vi "Bertta_v09_9.vi"() -> ()   [LabVIEW 2015]
panel:
  out "element":bool
  out "Started:":string
  in  "SHUTDOWN":bool
  in  "MASTER CONTROL":bool
  in  "Tab Control":T1(tab)
  out "Output File":path caption="selected path"
  in  "Browse folder":path=path "" caption="start path"
  in  "Read Seq":bool
  in  "Save Seq":bool
  in  "Configuration file":path=path "C:/Users/shresplab/Desktop/BerttaConfiguration.lvm" caption="Filename"
  in  "OK Button 2":bool
  out "Boolean":bool
  in  "User (initials)":string
  in  "Project name":string
  in  "Description":string
  out "PUMP1":bool
  out "Target amount":dbl
  out "Scale weight":dbl
  out "Amount now":dbl
  out "Flow rate":dbl
  out "Time to target":dbl format="%<%H:%M:%S>t"
  out "Current step":dbl
  out "Target":dbl
  out "Amount now":dbl
  out "Amount now":dbl
  out "Target":dbl
  out "Current step":dbl
  out "Time to target":dbl format="%<%H:%M:%S>t"
  out "Flow rate":dbl
  out "Amount now":dbl
  out "Scale weight":dbl
  out "Target amount":dbl
  out "PUMP2":bool
  out "Sensor OK 6":bool
  out "Sensor OK 5":bool
  out "Sensor OK 4":bool
  out "Sensor OK 3":bool
  in  "OK Button":bool
  in  "Add comment":string
  out "PUMP3":bool
  out "Target amount":dbl
  out "Scale weight":dbl
  out "Amount now":dbl
  out "Flow rate":dbl
  out "Time to target":dbl format="%<%H:%M:%S>t"
  out "Current step":dbl
  out "Target":dbl
  out "Amount now":dbl
  out "Tr":dbl
  out "Tj in":dbl
  out "Tj out":dbl
  out "T set":dbl
  out "Current step":i32
  out "RPM":dbl
  out "Torque 2":dbl
  out "Waveform Chart 5":dynamicdata(graph)
  out "Waveform Chart 6":dynamicdata(graph)
  out "Waveform Chart 7":dynamicdata(graph)
  in  "Tab Control 2":T2(tab)
  out "Waveform Chart 3":dynamicdata(graph)
  out "Waveform Chart 8":dynamicdata(graph)
  out "Waveform Chart 11":dynamicdata(graph)
  out "Waveform Chart 13":dynamicdata(graph)
  out "Waveform Chart 9":dynamicdata(graph)
  out "Table":string[][](table)=[["14.8.2017 18.06.59", "0,000000", "417,670000", "-0,150000", "1,000000", "22,220000", "23,366837", "23,574959", "23,985852", "23,690000", "240,000000", "4,000000", "0,000000", "397,000000", "-397,000000", "1,000000"], ["14.8.2017 18.07.06", "0,000000", "417,640000", "-0,120000", "1,000000", "22,220000", "23,763115", "23,906257", "23,985694", "23,680000", "240,000000", "4,000000", "0,000000", "397,000000", "-397,000000", "1,000000"], ["14.8.2017 18.07.13", "0,000000", "417,640000", "-0,120000", "1,000000", "22,220000", "23,965922", "24,013440", "23,984906", "23,670000", "240,000000", "4,100000", "3,000000", "397,000000", "-397,000000", "1,000000"], ["14.8.2017 18.07.21", "0,000000", "417,640000", "-0,120000", "1,000000", "22,220000", "23,943860", "23,900110", "23,987113", "23,670000", "240,000000", "4,000000", "0,000000", "397,000000", "-397,000000", "1,000000"], ["14.8.2017 18.07.28", "0,000000", "417,640000", "-0,120000", "1,000000", "22,220000", "23,736328", "23,600018", "23,989004", "23,660000", "240,000000", "4,000000", "0,000000", "397,000000", "-397,000000", "1,000000"], ["14.8.2017 18.07.36", "0,000000", "417,640000", "-0,120000", "1,000000", "22,220000", "23,480910", "23,324538", "23,991053", "23,660000", "240,000000", "4,000000", "0,000000", "397,000000", "-397,000000", "1,000000"], ["14.8.2017 18.07.43", "0,000000", "417,640000", "-0,120000", "2,000000", "22,220000", "23,195579", "23,008270", "23,999093", "23,650000", "240,000000", "4,000000", "0,000000", "397,000000", "-397,000000", "1,000000"], ["14.8.2017 18.07.51", "0,000000", "417,650000", "-417,650000", "1,000000", "22,220000", "22,862541", "22,649021", "24,003979", "23,650000", "240,000000", "4,000000", "0,000000", "397,000000", "-397,000000", "2,000000"], ["14.8.2017 18.07.58", "0,000000", "417,640000", "0,010000", "1,000000", "22,220000", "22,541353", "22,354878", "24,005398", "23,650000", "240,000000", "4,000000", "0,000000", "397,000000", "-397,000000", "1,000000"], ["14.8.2017 18.08.06", "0,000000", "417,640000", "0,010000", "1,000000", "22,220000", "22,347931", "22,253738", "24,007605", "23,640000", "240,000000", "4,100000", "0,000000", "397,000000", "-397,000000", "1,000000"], ["14.8.2017 18.08.13", "0,000000", "417,640000", "0,010000", "1,000000", "22,220000", "22,329030", "22,302102", "24,006028", "23,640000", "240,000000", "4,000000", "0,000000", "395,820000", "-395,820000", "1,000000"], ["14.8.2017 18.08.20", "0,000000", "417,640000", "0,010000", "1,000000", "22,220000", "22,466849", "22,511320", "24,002403", "23,630000", "240,000000", "4,000000", "0,000000", "395,830000", "-0,010000", "1,000000"], ["14.8.2017 18.08.28", "0,000000", "417,640000", "0,010000", "1,000000", "22,220000", "22,707062", "22,835101", "24,000984", "23,620000", "240,000000", "4,000000", "0,000000", "395,830000", "-0,010000", "1,000000"], ["14.8.2017 18.08.35", "0,000000", "417,640000", "0,010000", "1,000000", "22,220000", "23,054104", "23,232979", "24,001299", "23,600000", "240,000000", "4,000000", "0,000000", "395,830000", "-0,010000", "1,000000"], ["14.8.2017 18.08.43", "0,000000", "417,640000", "0,010000", "1,000000", "22,220000", "23,412371", "23,522793", "24,002560", "23,590000", "240,000000", "4,000000", "0,000000", "395,820000", "0,000000", "1,000000"], ["14.8.2017 18.08.51", "0,000000", "417,640000", "0,010000", "1,000000", "22,220000", "23,596247", "23,656125", "24,003821", "23,580000", "240,000000", "4,000000", "0,000000", "395,820000", "0,000000", "1,000000"]]
  in  "Time":dbl
  out "Current temp":dbl
  in  "OK Button 3":bool
  in  "Reset":bool
  in  "Temp5":dbl=20.0
  in  "Temp4":dbl=30.0
  in  "Temp3":dbl=40.0
  in  "Temp2":dbl=30.0
  in  "Temp1":dbl=20.0
  out "Boolean 12":bool
  out "Boolean 7":bool
  out "Boolean 6":bool
  out "Boolean 5":bool
  out "Boolean 4":bool
  out "Boolean 19":bool
  in  "Time1":dbl=5.0
  in  "Time2":dbl=5.0
  in  "Time3":dbl=5.0
  in  "Time4":dbl=5.0
  in  "T ext / T ext 2":enum32{"External 1", "External 2"}(radio)
  out "Sensor OK":bool
  in  "T fail":dbl=20.0
  in  "?":bool
  in  "Setpoint":dbl=20.0
  in  "Manual select":enum32{"Tr", "Tj"}(radio)
  in  "PAUSE":bool
  out "Waveform Chart":dynamicdata(graph)
  out "T external 2":dbl
  out "Led11 5":bool
  out "RPM":dbl format="%_4f"
  out "Led10 3":bool
  out "Led9 3":bool
  out "Led8 3":bool
  out "Led7 3":bool
  out "Led6 3":bool
  out "Led5 3":bool
  out "Led4 3":bool
  out "Led3 3":bool
  out "Led2 3":bool
  out "Led1 3":bool
  in  "PumpSeq 4":dbl[][](array[numeric])=[[1.0, 1.0, 0.0, 0.0, 0.0, 0.0, 0.0, 0.0, 0.0, 0.0], [2.0, 1.0, 0.0, 0.0, 0.0, 0.0, 0.0, 0.0, 0.0, 0.0], [3.0, 1.0, 0.0, 0.0, 0.0, 0.0, 0.0, 0.0, 0.0, 0.0], [0.0, 0.0, 0.0, 0.0, 0.0, 0.0, 0.0, 0.0, 0.0, 0.0], [0.0, 0.0, 0.0, 0.0, 0.0, 0.0, 0.0, 0.0, 0.0, 0.0], [0.0, 0.0, 0.0, 0.0, 0.0, 0.0, 0.0, 0.0, 0.0, 0.0], [0.0, 0.0, 0.0, 0.0, 0.0, 0.0, 0.0, 0.0, 0.0, 0.0], [0.0, 0.0, 0.0, 0.0, 0.0, 0.0, 0.0, 0.0, 0.0, 0.0], [0.0, 0.0, 0.0, 0.0, 0.0, 0.0, 0.0, 0.0, 0.0, 0.0], [0.0, 0.0, 0.0, 0.0, 0.0, 0.0, 0.0, 0.0, 0.0, 0.0]]
  in  "?":bool
  out "Flow rate (g/min)":dbl
  out "Scale reading":dbl
  out "Step amount now":dbl
  in  "Grams / min":dbl
  out "Waveform Chart 14":dynamicdata(graph)
  in  "?":bool
  out "Total amount now":dbl
  out "Led11 4":bool
  in  "Reset 5":bool
  out "Elapsed / step":i32
  out "Time to target":dbl format="%<%H:%M:%S>t"
  in  "OK Button 4":bool
  out "Led11":bool
  out "RPM":dbl format="%_4f"
  out "Led10":bool
  out "Led9":bool
  out "Led8":bool
  out "Led7":bool
  out "Led6":bool
  out "Led5":bool
  out "Led4":bool
  out "Led3":bool
  out "Led2":bool
  out "Led1":bool
  in  "PumpSeq 2":dbl[][](array[numeric])=[[1.0, 2.0, 0.0, 0.0, 0.0, 0.0, 0.0, 0.0, 0.0, 0.0], [2.0, 2.0, 0.0, 0.0, 0.0, 0.0, 0.0, 0.0, 0.0, 0.0], [3.0, 2.0, 0.0, 0.0, 0.0, 0.0, 0.0, 0.0, 0.0, 0.0], [0.0, 0.0, 0.0, 0.0, 0.0, 0.0, 0.0, 0.0, 0.0, 0.0], [0.0, 0.0, 0.0, 0.0, 0.0, 0.0, 0.0, 0.0, 0.0, 0.0], [0.0, 0.0, 0.0, 0.0, 0.0, 0.0, 0.0, 0.0, 0.0, 0.0], [0.0, 0.0, 0.0, 0.0, 0.0, 0.0, 0.0, 0.0, 0.0, 0.0], [0.0, 0.0, 0.0, 0.0, 0.0, 0.0, 0.0, 0.0, 0.0, 0.0], [0.0, 0.0, 0.0, 0.0, 0.0, 0.0, 0.0, 0.0, 0.0, 0.0], [0.0, 0.0, 0.0, 0.0, 0.0, 0.0, 0.0, 0.0, 0.0, 0.0]]
  in  "?":bool
  out "Flow rate (g/min)":dbl
  out "Scale reading":dbl
  out "Step amount now":dbl
  in  "Grams / min":dbl
  out "Waveform Chart 10":dynamicdata(graph)
  in  "?":bool
  out "Total amount now":dbl
  out "Led11":bool
  in  "Reset 3":bool
  out "Elapsed / step":i32
  out "Time to target":dbl format="%<%H:%M:%S>t"
  in  "OK Button 5":bool
  out "Led11 3":bool
  out "RPM":dbl format="%_4f"
  out "Led10 2":bool
  out "Led9 2":bool
  out "Led8 2":bool
  out "Led7 2":bool
  out "Led6 2":bool
  out "Led5 2":bool
  out "Led4 2":bool
  out "Led3 2":bool
  out "Led2 2":bool
  out "Led1 2":bool
  in  "PumpSeq 3":dbl[][](array[numeric])=[[1.0, 3.0, 0.0, 0.0, 0.0, 0.0, 0.0, 0.0, 0.0, 0.0], [2.0, 3.0, 0.0, 0.0, 0.0, 0.0, 0.0, 0.0, 0.0, 0.0], [3.0, 3.0, 0.0, 0.0, 0.0, 0.0, 0.0, 0.0, 0.0, 0.0], [0.0, 0.0, 0.0, 0.0, 0.0, 0.0, 0.0, 0.0, 0.0, 0.0], [0.0, 0.0, 0.0, 0.0, 0.0, 0.0, 0.0, 0.0, 0.0, 0.0], [0.0, 0.0, 0.0, 0.0, 0.0, 0.0, 0.0, 0.0, 0.0, 0.0], [0.0, 0.0, 0.0, 0.0, 0.0, 0.0, 0.0, 0.0, 0.0, 0.0], [0.0, 0.0, 0.0, 0.0, 0.0, 0.0, 0.0, 0.0, 0.0, 0.0], [0.0, 0.0, 0.0, 0.0, 0.0, 0.0, 0.0, 0.0, 0.0, 0.0], [0.0, 0.0, 0.0, 0.0, 0.0, 0.0, 0.0, 0.0, 0.0, 0.0]]
  in  "?":bool
  out "Flow rate (g/min)":dbl
  out "Scale reading":dbl
  out "Step amount now":dbl
  in  "Grams / min":dbl
  out "Waveform Chart 12":dynamicdata(graph)
  in  "?":bool
  out "Total amount now":dbl
  out "Led11 2":bool
  in  "Reset 4":bool
  out "Elapsed / step":i32
  out "Time to target":dbl format="%<%H:%M:%S>t"
  in  "OK Button 6":bool
  in  "Bypass select 2":enum32{"Remote", "Manual"}(radio)=enum."Manual"
  in  "Port":dbl=13.0
  out "RPM":dbl
  out "Torque":dbl
  in  "Set RPM":dbl(slide) scale=0.0..2000.0
  out "Waveform Chart 4":dynamicdata(graph)
  in  "OK Button 7":bool
  in  "Treshold (T/C)":dbl=0.5
  out "DAQ 9217 (PT100)":errorcluster
  out "Config File":dbl[][](array[numeric])
  # "Temperature sensor:"
  # "Manual control:"
  # "PUMP & SCALE 1"
  # "STEP"
  # "TOTAL"
  # "PUMP & SCALE 2"
  # "STEP"
  # "TOTAL"
  # "PUMP & SCALE 3"
  # "STEP"
  # "TOTAL"
  # "Manual temperature control"
  # "Secondary temperature sensor"
  # "Temp"
  # "Time"
  # "Grams    /   min"
  # "End of sequence"
  # "Manual control"
  # "Grams    /   min"
  # "End of sequence"
  # "Manual control"
  # "Grams    /   min"
  # "End of sequence"
  # "Manual control"
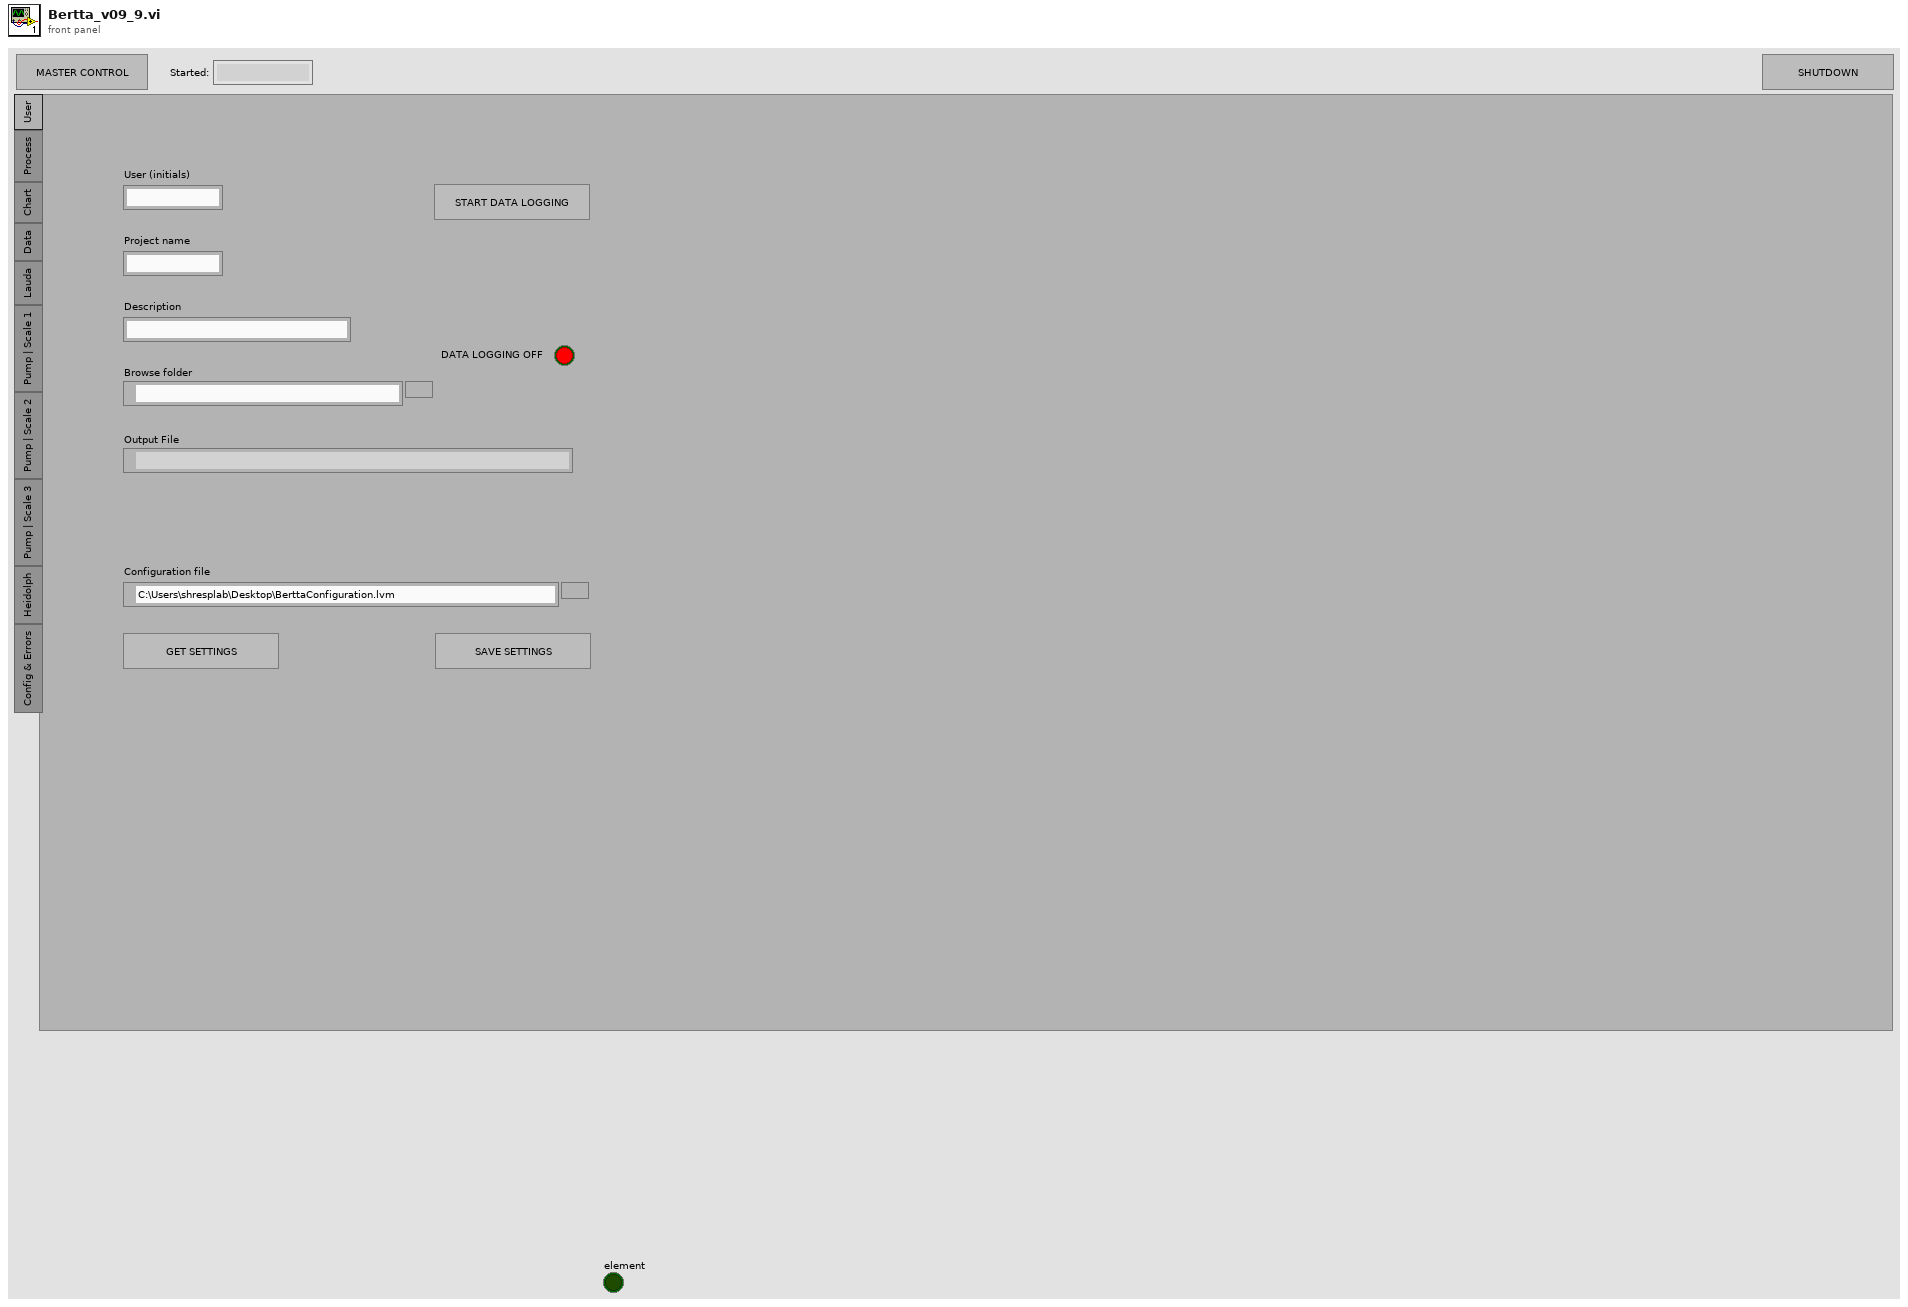
[diagram p1: front panel]
types:
  T1 = enum32{"User", "Process", "Chart", "Data", "Lauda", "Pump | Scale 1", "Pump | Scale 2", "Pump | Scale 3", "Heidolph", "Config & Errors"}
  T2 = enum32{"Temperatures", "Scale / Pump 1", "Scale / Pump 2", "Scale / Pump 3", "RPM / torque"}
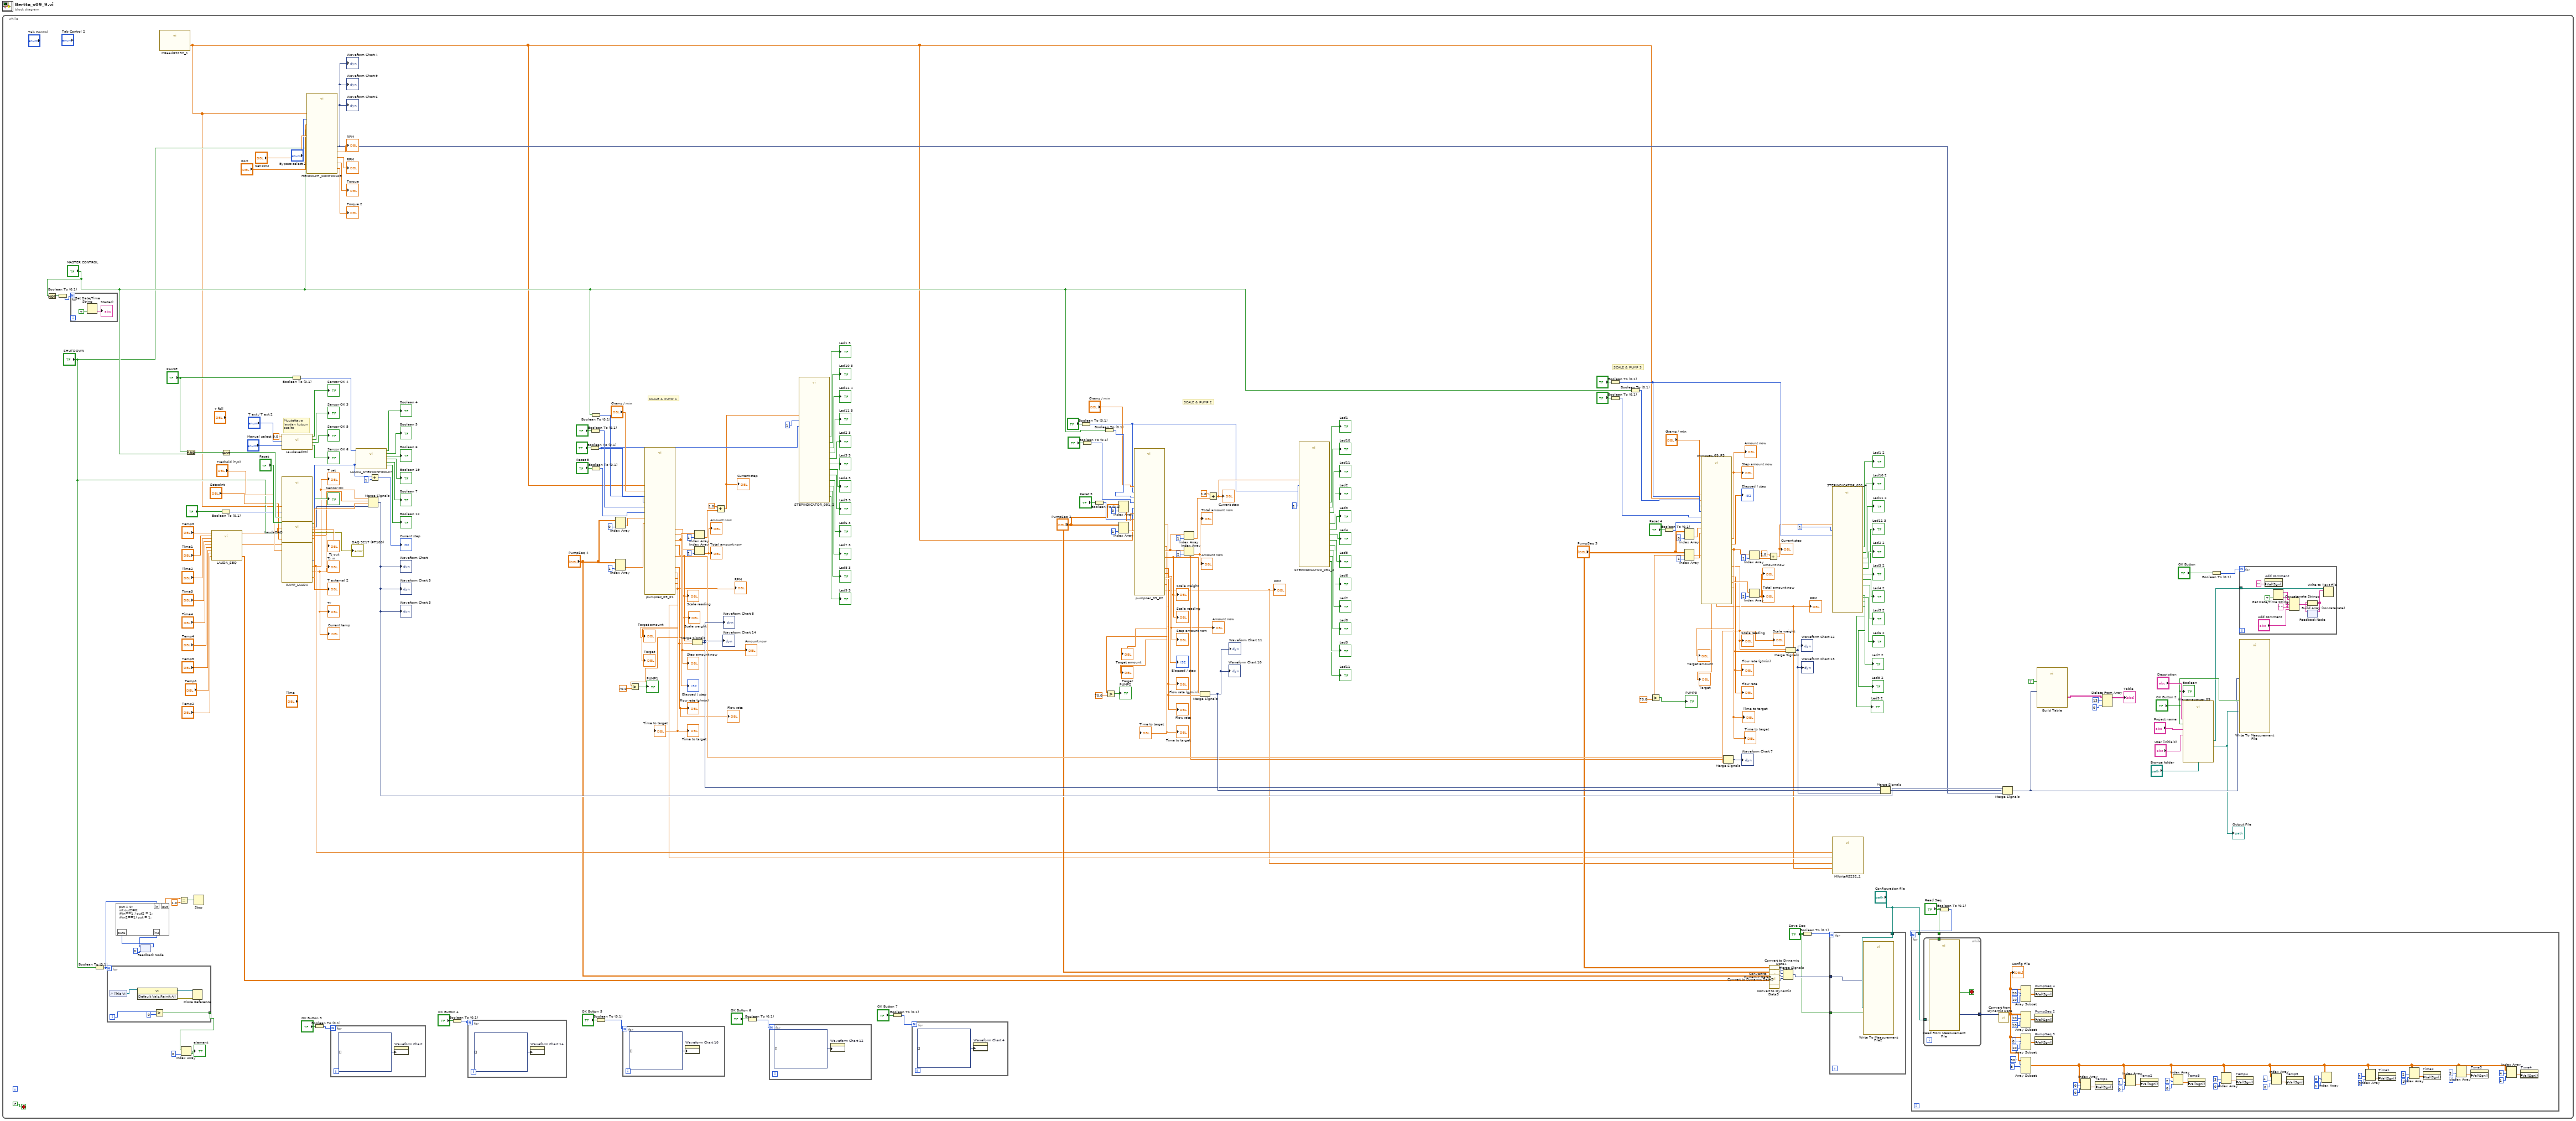
[diagram p0: block diagram]
diagram:
  n1 = while {
    stop <- FALSE stop-if-true
    # "Muutettava\nlaudan kutsun \nosalta"
    # "SCALE & PUMP 1"
    # "SCALE & PUMP 3"
    # "SCALE & PUMP 2"
    n2 = Not(x="MASTER CONTROL") -> (.not. x?=w226:bool)
    n3 = Boolean To (0,1)(Boolean=w226) -> (0, 1=w227:i16)
    n4 = for {
      N: w227 -> [_]
      n5 = Get Date/Time String(want seconds? (F)=TRUE) -> (time string=→"Started:":string)  [unwired: 2 in, 1 out]
    }
    n6 = Boolean To (0,1)(Boolean="SHUTDOWN") -> (0, 1=w209:i16)
    n7 = for {
      N: w209 -> [_]
      tunnel: [w311] -> w225 mode=indexing
      i -> [w313]
      n8 = control-ref of="This VI"() -> (w316:refnum<vi>)
      n9 = invoke class="VI" method="Default Vals.Reinit All"(reference=w316) -> (reference out=w314:refnum<vi>, error out=w315:errorcluster)  [unwired: 2 in, 1 out]
      n10 = Greater?(x=w313, y=0) -> (0:w311:bool)
      n11 = Close Reference(reference=w314, error in (no error)=w315) -> ()  [unwired: 1 out]
    }
    n12 = feedback #1(0) -> (w207:i32)
    n13 = formula code="out = 0;\nint out2=0;\nif(in==1 ) out2 = 1;\nif(in2==1) out = 1;"("in"=w209, "in2"=w207) -> ("out"=w211:dbl, "out2"=w208:i32)
    n14 = feedback-in #1(w208) -> ()
    n15 = call "MReadRS232_1.vi"() -> ("params"=w21:dbl[])  [unwired: 11 in]
    n16 = Equal?(x=w211, y=1.0) -> (x = y?=w210:bool)
    n17 = Index Array(array=w225, index=0) -> (element=→"element":bool)
    n18 = And(x="PAUSE", y="MASTER CONTROL") -> (x .and. y?=w171:bool)
    n19 = Stop(stop? (T)=w210) -> ()
    n20 = call "LAUDA_SEQ.vi"("Numeric 2"="Temp3", "Numeric 1"="Temp2", "Numeric"="Temp1", "Numeric 5"="Time1", "Numeric 6"="Time2", "Numeric 7"="Time3", "Numeric 8"="Time4", "Numeric 3"="Temp4", "Numeric 4"="Temp5") -> ("output array"=w26:dbl[], "output array 2"=w27:dbl[], "appended array"=w25:dbl[][])  [unwired: 4 in]
    n21 = Boolean To (0,1)(Boolean="?") -> (0, 1=w158:i16)
    n22 = Not(x=w171) -> (.not. x?=w170:bool)
    n23 = call "LaudaLedCtrl.vi"("Manual select"="Manual select", "T ext / T ext in"="T ext / T ext 2", "Lauda port"=9.0) -> ("Sensor OK 5"=→"Sensor OK 5":bool, "Sensor OK 3"=→"Sensor OK 3":bool, "Sensor OK 4"=→"Sensor OK 4":bool, "Sensor OK 6"=→"Sensor OK 6":bool)  [unwired: 5 in]
    n24 = call "RAMP_LAUDA.vi"("pause"=w170, "manual"=w158, "Array"=w21, "T_man"="Setpoint", "Seq"=w26, "reset"="Reset", "TimeParams"=w27, "shutdown"="SHUTDOWN", "treshold"="Treshold (T/C)") -> ("T in"=w80:dbl, "STEP"=w50:i32, "T ext"=w1:dbl, "T control"=w20:dbl)  [unwired: 2 in, 1 out]
    "Tr" <- w1
    "T set" <- w20
    "Current temp" <- w1
    n25 = call "LaudaDAQ.vi"() -> ("error out"=→"DAQ 9217 (PT100)":errorcluster, 1:"Tj out"=→"Tj out":dbl, "data"=w79:dynamicdata, "Sensor OK"=→"Sensor OK":bool, 4:"Tj out"=→"Tj in":dbl, "T external 2"=→"T external 2":dbl)  [unwired: 6 in]
    n26 = Boolean To (0,1)(Boolean="PAUSE") -> (0, 1=w204:i16)
    n27 = call "HEIDOLPH_CONTROL09.vi"("master"="MASTER CONTROL", "Array"=w21, "shutdown"="SHUTDOWN", "Bypass select"="Bypass select 2", "Set RPM"="Set RPM", "Device port"="Port") -> ("Dynamic Data"=w81:dynamicdata, "RPM"=→"RPM":dbl, "RPM 2"=→"RPM":dbl, "Torque"=→"Torque":dbl, "Torque 2"=→"Torque 2":dbl)  [unwired: 1 in]
    "Waveform Chart 4" <- w81
    "Waveform Chart 6" <- w81
    "Waveform Chart 9" <- w81
    n28 = Boolean To (0,1)(Boolean="OK Button 3") -> (0, 1=w12:i16)
    n29 = for {
      N: w12 -> [_]
      n30 = property on="Waveform Chart" class="WFChart (strict)"("History Data"=dynamicdata[] []) -> ()  [unwired: 2 in, 2 out]
    }
    n31 = call "LAUDA_STEPCONTROL07.vi"("step"=w50, "pause"=w204) -> ("Boolean 13"=→"Boolean 19":bool, "Boolean 6"=→"Boolean 6":bool, "Boolean 5"=→"Boolean 5":bool, "Boolean 4"=→"Boolean 4":bool, "Boolean 7"=→"Boolean 7":bool, "Boolean 12"=→"Boolean 12":bool)  [unwired: 4 in]
    n32 = Merge Signals(w20, w1, w80, w79) -> (w82:dynamicdata)
    "Waveform Chart 3" <- w82
    "Waveform Chart" <- w82
    "Waveform Chart 5" <- w82
    n33 = Add(x=w50, y=1) -> (x+y=→"Current step":i32)
    n34 = Boolean To (0,1)(Boolean="OK Button 4") -> (0, 1=w10:i16)
    n35 = for {
      N: w10 -> [_]
      n36 = property on="Waveform Chart 14" class="WFChart (strict)"("History Data"=dynamicdata[] []) -> ()  [unwired: 2 in, 2 out]
    }
    n37 = Boolean To (0,1)(Boolean="?") -> (0, 1=w91:i16)
    n38 = Boolean To (0,1)(Boolean="?") -> (0, 1=w95:i16)
    n39 = Boolean To (0,1)(Boolean="MASTER CONTROL") -> (0, 1=w87:i16)
    n40 = Boolean To (0,1)(Boolean="Reset 5") -> (0, 1=w94:i16)
    n41 = Boolean To (0,1)(Boolean="OK Button 5") -> (0, 1=w8:i16)
    n42 = Index Array(array="PumpSeq 4", index (col)=0) -> (element=w99:dbl[])  [unwired: 1 in]
    n43 = Index Array(array="PumpSeq 4", index (col)=1) -> (element=w120:dbl[])  [unwired: 1 in]
    n44 = for {
      N: w8 -> [_]
      n45 = property on="Waveform Chart 10" class="WFChart (strict)"("History Data"=dynamicdata[] []) -> ()  [unwired: 2 in, 2 out]
    }
    n46 = call "pumpsec_09_P1.vi"("reset"=w94, "master"=w87, "manual"=w91, "pause"=w95, "Array"=w21, "Target"=w99, "fr_manual"="Grams / min", "Time"=w120) -> ("pumpCtrl"=w63:dbl, "totaltarget"=→"Target":dbl, "target_step"=→"Target amount":dbl, "REGLO D"=w19:dbl, "time_to_target"=→"Time to target" →"Time to target":dbl, "step_fr"=w36:dbl, "amount_step"=→"Amount now" →"Step amount now":dbl, "Scale"=w75:dbl, "elapsed_step"=→"Elapsed / step":dbl, "params"=w117:dbl[])  [unwired: 8 in, 2 out]
    "Flow rate" <- w36
    "Scale weight" <- w75
    "Scale reading" <- w75
    "Flow rate (g/min)" <- w36
    "RPM" <- w19
    n47 = Greater?(x=w63, y=70.0) -> (0:→"PUMP1":bool)
    n48 = Merge Signals(w75, w36) -> (w85:dynamicdata)
    "Waveform Chart 8" <- w85
    "Waveform Chart 14" <- w85
    n49 = Index Array(array=w117, index=1) -> (element=w114:dbl)
    n50 = Index Array(array=w117, index=2) -> (element=→"Amount now" →"Total amount now":dbl)
    n51 = Add(x=1.0, y=w114) -> (x+y=w37:dbl)
    "Current step" <- w37
    n52 = Boolean To (0,1)(Boolean="OK Button 6") -> (0, 1=w6:i16)
    n53 = for {
      N: w6 -> [_]
      n54 = property on="Waveform Chart 12" class="WFChart (strict)"("History Data"=dynamicdata[] []) -> ()  [unwired: 2 in, 2 out]
    }
    n55 = call "STEPINDICATOR_091_2.vi"("current step"=w37, "enable"=i16 1, "manual"=w91) -> ("Led 8"=→"Led8 3":bool, "Led 10"=→"Led10 3":bool, "Led 11"=→"Led11 4":bool, "Led 7"=→"Led7 3":bool, "Led 1"=→"Led1 3":bool, "Led 6"=→"Led6 3":bool, "Led 2"=→"Led2 3":bool, "Led 12"=→"Led11 5":bool, "Led 5"=→"Led5 3":bool, "Led 4"=→"Led4 3":bool, "Led 3"=→"Led3 3":bool, "Led 9"=→"Led9 3":bool)  [unwired: 1 in]
    n56 = Boolean To (0,1)(Boolean="OK Button 7") -> (0, 1=w4:i16)
    n57 = for {
      N: w4 -> [_]
      n58 = property on="Waveform Chart 4" class="WFChart (strict)"("History Data"=dynamicdata[] []) -> ()  [unwired: 2 in, 2 out]
    }
    n59 = Boolean To (0,1)(Boolean="?") -> (0, 1=w154:i16)
    n60 = Boolean To (0,1)(Boolean="?") -> (0, 1=w197:i16)
    n61 = Boolean To (0,1)(Boolean="Reset 3") -> (0, 1=w195:i16)
    n62 = Boolean To (0,1)(Boolean="MASTER CONTROL") -> (0, 1=w189:i16)
    n63 = Index Array(array="PumpSeq 2", index (col)=0 ("disabled index (col)")) -> (element=w200:dbl[])  [unwired: 1 in]
    n64 = Index Array(array="PumpSeq 2", index (col)=1 ("disabled index (col)")) -> (element=w199:dbl[])  [unwired: 1 in]
    n65 = call "pumpsec_09_P2.vi"("reset"=w195, "master"=w189, "manual"=w154, "pause"=w197, "Array"=w21, "Target"=w200, "fr_manual"="Grams / min", "Time"=w199) -> ("pumpCtrl"=w59:dbl, "totaltarget"=→"Target":dbl, "target_step"=→"Target amount":dbl, "REGLO D"=w18:dbl, "time_to_target"=→"Time to target" →"Time to target":dbl, "step_fr"=w78:dbl, "amount_step"=→"Amount now" →"Step amount now":dbl, "Scale"=w74:dbl, "elapsed_step"=→"Elapsed / step":dbl, "params"=w190:dbl[])  [unwired: 8 in, 2 out]
    "Scale weight" <- w74
    "Flow rate" <- w78
    "Scale reading" <- w74
    "Flow rate (g/min)" <- w78
    "RPM" <- w18
    n66 = Greater?(x=w59, y=70.0) -> (0:→"PUMP2":bool)
    n67 = Index Array(array=w190, index=1) -> (element=w193:dbl)
    n68 = Index Array(array=w190, index=2) -> (element=→"Amount now" →"Total amount now":dbl)
    n69 = Merge Signals(w74, w78) -> (w88:dynamicdata)
    "Waveform Chart 11" <- w88
    "Waveform Chart 10" <- w88
    n70 = Add(x=1.0, y=w193) -> (x+y=w187:dbl)
    "Current step" <- w187
    n71 = call "STEPINDICATOR_091_2.vi"("current step"=w187, "enable"=i16 1, "manual"=w154) -> ("Led 8"=→"Led8":bool, "Led 10"=→"Led10":bool, "Led 11"=→"Led11":bool, "Led 7"=→"Led7":bool, "Led 1"=→"Led1":bool, "Led 6"=→"Led6":bool, "Led 2"=→"Led2":bool, "Led 12"=→"Led11":bool, "Led 5"=→"Led5":bool, "Led 4"=→"Led4":bool, "Led 3"=→"Led3":bool, "Led 9"=→"Led9":bool)  [unwired: 1 in]
    n72 = Boolean To (0,1)(Boolean="?") -> (0, 1=w148:i16)
    n73 = Boolean To (0,1)(Boolean="?") -> (0, 1=w147:i16)
    n74 = Boolean To (0,1)(Boolean="MASTER CONTROL") -> (0, 1=w149:i16)
    n75 = Boolean To (0,1)(Boolean="Reset 4") -> (0, 1=w129:i16)
    n76 = Index Array(array="PumpSeq 3", index (col)=0 ("disabled index (col)")) -> (element=w132:dbl[])  [unwired: 1 in]
    n77 = Index Array(array="PumpSeq 3", index (col)=1 ("disabled index (col)")) -> (element=w131:dbl[])  [unwired: 1 in]
    n78 = call "pumpsec_09_P3.vi"("reset"=w129, "master"=w149, "manual"=w148, "pause"=w147, "Array"=w21, "Target"=w132, "fr_manual"="Grams / min", "Time"=w131) -> ("pumpCtrl"=w56:dbl, "totaltarget"=→"Target":dbl, "target_step"=→"Target amount":dbl, "REGLO D"=w17:dbl, "time_to_target"=→"Time to target" →"Time to target":dbl, "step_fr"=w77:dbl, "amount_step"=→"Amount now" →"Step amount now":dbl, "Scale"=w73:dbl, "elapsed_step"=→"Elapsed / step":dbl, "params"=w122:dbl[])  [unwired: 8 in, 2 out]
    "Scale weight" <- w73
    "Flow rate" <- w77
    "Scale reading" <- w73
    "Flow rate (g/min)" <- w77
    "RPM" <- w17
    n79 = Greater?(x=w56, y=70.0) -> (0:→"PUMP3":bool)
    n80 = Merge Signals(w75, w74, w73) -> (→"Waveform Chart 7":dynamicdata)
    n81 = Index Array(array=w122, index=1) -> (element=w123:dbl)
    n82 = Index Array(array=w122, index=2) -> (element=→"Amount now" →"Total amount now":dbl)
    n83 = Add(x=1.0, y=w123) -> (x+y=w121:dbl)
    "Current step" <- w121
    n84 = call "Convert to Dynamic Data4"("2D Array"="PumpSeq 3") -> ("Dynamic Data Type"=w28:dynamicdata)  [unwired: 3 in]
    n85 = call "Convert to Dynamic Data3"("2D Array"="PumpSeq 2") -> ("Dynamic Data Type"=w30:dynamicdata)  [unwired: 3 in]
    n86 = call "Convert to Dynamic Data2"("2D Array"="PumpSeq 4") -> ("Dynamic Data Type"=w33:dynamicdata)  [unwired: 3 in]
    n87 = call "Convert to Dynamic Data5"("2D Array"=w25) -> ("Dynamic Data Type"=w24:dynamicdata)  [unwired: 3 in]
    n88 = Merge Signals(w28, w30, w33, w24) -> (w32:dynamicdata)
    n89 = Merge Signals(w73, w77) -> (w84:dynamicdata)
    "Waveform Chart 13" <- w84
    "Waveform Chart 12" <- w84
    n90 = Boolean To (0,1)(Boolean="Save Seq") -> (0, 1=w23:i16)
    n91 = for {
      N: w23 -> [_]
      tunnel: w32 -> [w309]
      tunnel: "Configuration file" -> [w310]
      tunnel: "Save Seq" -> [w308]
      n92 = call "Write To Measurement File2"("Signals"=w309, "Reset"=w308, "Filename"=w310) -> ()  [unwired: 14 in, 3 out]
    }
    n93 = call "STEPINDICATOR_091_4.vi"("current step"=w121, "enable"=i16 1, "manual"=w148) -> ("Led 8"=→"Led8 2":bool, "Led 10"=→"Led10 2":bool, "Led 11"=→"Led11 2":bool, "Led 7"=→"Led7 2":bool, "Led 1"=→"Led1 2":bool, "Led 6"=→"Led6 2":bool, "Led 2"=→"Led2 2":bool, "Led 12"=→"Led11 3":bool, "Led 5"=→"Led5 2":bool, "Led 4"=→"Led4 2":bool, "Led 3"=→"Led3 2":bool, "Led 9"=→"Led9 2":bool)  [unwired: 1 in]
    n94 = call "MWriteRS232_1.vi"("P3"=w17, "P2"=w18, "P1"=w19, "LAUDA"=w20) -> ()  [unwired: 8 in]
    n95 = Merge Signals(w85, w88, w84) -> (w83:dynamicdata)
    n96 = Boolean To (0,1)(Boolean="Read Seq") -> (0, 1=w22:i16)
    n97 = for {
      N: w22 -> [_]
      tunnel: "Configuration file" -> [w260]
      tunnel: "Read Seq" -> [w259]
      n98 = while {
        tunnel: [w307] -> w303
        tunnel: w260 -> [w306]
        tunnel: w259 -> [w304]
        stop <- w305 stop-if-true
        n99 = call "Read From Measurement File"("Filename"=w306, "Reset"=w304) -> ("Signals"=w307:dynamicdata, "EOF?"=w305:bool)  [unwired: 4 in, 4 out]
      }
      n100 = call "Convert from Dynamic Data"("Dynamic Data Type"=w303) -> ("Array"=w293:dbl[][])  [unwired: 3 in]
      "Config File" <- w293
      n101 = Array Subset(array=w293, index (row)=20 ("index"), length (row)=10 ("length")) -> (w300:dbl[][])  [unwired: 2 in]
      n102 = Array Subset(array=w293, index (row)=10 ("index"), length (row)=10 ("length")) -> (w295:dbl[][])  [unwired: 2 in]
      n103 = Array Subset(array=w293, index (row)=0 ("index"), length (row)=10 ("length")) -> (w294:dbl[][])  [unwired: 2 in]
      n104 = Array Subset(array=w293, index (row)=30 ("index"), length (row)=8 ("length")) -> (w270:dbl[][])  [unwired: 2 in]
      n105 = property on="PumpSeq 4" class="Arr (strict)"("Val(Sgnl)"=w300) -> ()  [unwired: 2 in, 2 out]
      n106 = property on="PumpSeq 2" class="Arr (strict)"("Val(Sgnl)"=w295) -> ()  [unwired: 2 in, 2 out]
      n107 = property on="PumpSeq 3" class="Arr (strict)"("Val(Sgnl)"=w294) -> ()  [unwired: 2 in, 2 out]
      n108 = Index Array(array=w270, index (row)=0, index (col)=0 ("disabled index (col)")) -> (element=w269:dbl)
      n109 = property on="Temp1" class="DigNum (strict)"("Val(Sgnl)"=w269) -> ()  [unwired: 2 in, 2 out]
      n110 = Index Array(array=w270, index (row)=1, index (col)=0 ("disabled index (col)")) -> (element=w268:dbl)
      n111 = property on="Temp2" class="DigNum (strict)"("Val(Sgnl)"=w268) -> ()  [unwired: 2 in, 2 out]
      n112 = Index Array(array=w270, index (row)=2, index (col)=0 ("disabled index (col)")) -> (element=w267:dbl)
      n113 = property on="Temp3" class="DigNum (strict)"("Val(Sgnl)"=w267) -> ()  [unwired: 2 in, 2 out]
      n114 = Index Array(array=w270, index (row)=3, index (col)=0 ("disabled index (col)")) -> (element=w266:dbl)
      n115 = property on="Temp4" class="DigNum (strict)"("Val(Sgnl)"=w266) -> ()  [unwired: 2 in, 2 out]
      n116 = Index Array(array=w270, index (row)=4, index (col)=0 ("disabled index (col)")) -> (element=w265:dbl)
      n117 = property on="Temp5" class="DigNum (strict)"("Val(Sgnl)"=w265) -> ()  [unwired: 2 in, 2 out]
      n118 = Index Array(array=w270, index (row)=0, index (col)=1 ("disabled index (col)")) -> ()  [unwired: 1 out]
      n119 = Index Array(array=w270, index (row)=1, index (col)=1 ("disabled index (col)")) -> (element=w264:dbl)
      n120 = property on="Time1" class="DigNum (strict)"("Val(Sgnl)"=w264) -> ()  [unwired: 2 in, 2 out]
      n121 = Index Array(array=w270, index (row)=2, index (col)=1 ("disabled index (col)")) -> (element=w263:dbl)
      n122 = property on="Time2" class="DigNum (strict)"("Val(Sgnl)"=w263) -> ()  [unwired: 2 in, 2 out]
      n123 = Index Array(array=w270, index (row)=3, index (col)=1 ("disabled index (col)")) -> (element=w262:dbl)
      n124 = property on="Time3" class="DigNum (strict)"("Val(Sgnl)"=w262) -> ()  [unwired: 2 in, 2 out]
      n125 = Index Array(array=w270, index (row)=4, index (col)=1 ("disabled index (col)")) -> (element=w261:dbl)
      n126 = property on="Time4" class="DigNum (strict)"("Val(Sgnl)"=w261) -> ()  [unwired: 2 in, 2 out]
    }
    n127 = Merge Signals(w82, w83, w81) -> (w220:dynamicdata)
    n128 = call "Build Table"("Include time data"=TRUE, "Signals"=w220) -> ("Table"=w219:string[][])  [unwired: 3 in, 6 out]
    n129 = Delete From Array(array=w219, length=13, index (col)=0 ("index (row)")) -> (array with subset deleted=→"Table":string[][])  [unwired: 1 in, 1 out]
    n130 = call "filenameparser_09.vi"("Description"="Description", "start path"="Browse folder", "Project name"="Project name", "User (initials)"="User (initials)", "OK Button in"="OK Button 2") -> ("appended path 2"=w2:path, "appended path"=w215:path)  [unwired: 4 in, 1 out]
    "Output File" <- w2
    n131 = Boolean To (0,1)(Boolean="OK Button") -> (0, 1=w214:i16)
    n132 = for {
      N: w214 -> [_]
      tunnel: w215 -> [w251]
      w255 = " " ("string")
      n133 = property on="Add comment" class="Str"("Val(Sgnl)"="" ("Value (Signaling)")) -> ()  [unwired: 2 in, 2 out]
      n134 = Get Date/Time String(want seconds? (F)=TRUE) -> (date string=w258:string, time string=w256:string)  [unwired: 2 in]
      n135 = Concatenate Strings(w258, w255, w256, w255, "Add comment") -> (w254:string)
      n136 = feedback #2() -> (w253:string[])  [unwired: 1 in]
      n137 = Build Array (concatenate)(w253, w254) -> (w252:string[])
      n138 = feedback-in #2(w252) -> ()
      n139 = Write to Text File(file (use dialog)=w251, text=w252) -> ()  [unwired: 2 in, 3 out]
    }
    n140 = call "Write To Measurement File"("Signals"=w220, "Enable"="OK Button 2", "Filename"=w2) -> ()  [unwired: 14 in, 3 out]
    "Boolean" <- "OK Button 2"
  }
